vi "Aquire Thermal Data.vi"(8 "error in (no error)":errorcluster, 10 "AI Aquisition Time(s)":dbl, 11 "Recipe Process in":refnum<class "Recipe Process.lvclass">) -> (0 "error out":errorcluster, 3 "Recipe Process out":refnum<class "Recipe Process.lvclass">)   [LabVIEW 2022 SP3, in "Recipe Process.lvlib" / "Recipe Process.lvclass"]
uses:
  Recipe Process.lvclass
  Recipe Process.lvclass/Recipe Process.ctl
  Camera/Camera Controller/Camera Controller.lvclass
  IO Monitor/DAQ API/DAQ API.lvclass
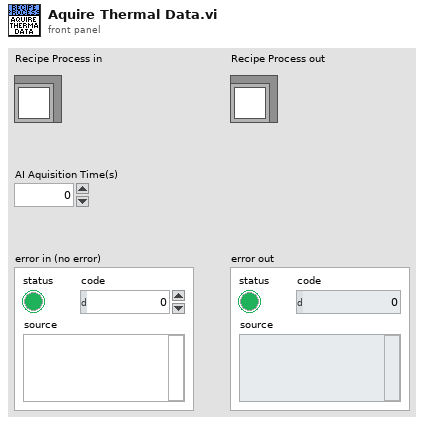
[diagram p1: front panel]
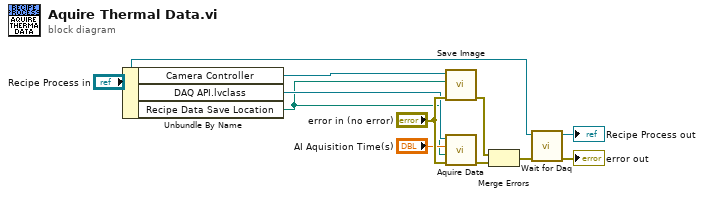
[diagram p0: block diagram]
diagram:
  n1 = Unbundle By Name("Recipe Process in") -> ("Camera Controller"=w2:refnum<class "Camera Controller.lvclass">, "DAQ API.lvclass"=w3:refnum<class "DAQ API.lvclass">, "Recipe Data Save Location"=w1:path)
  n2 = call-dynamic "Save Image.vi"("error in (no error)"="error in (no error)", "Path"=w1, "Camera Controller in"=w2) -> ("error out"=w6:errorcluster)  [unwired: 7 in, 1 out]
  n3 = call-dynamic "Aquire Data.vi"("error in (no error)"="error in (no error)", "Data Save Location"=w1, "Aqusition Time (s)"="AI Aquisition Time(s)", "Aquire Data in"=w3) -> ("error out"=w7:errorcluster)  [unwired: 6 in, 1 out]
  n4 = Merge Errors(w6, w7) -> (w9:errorcluster)
  n5 = call "Wait for Daq.vi"("error in (no error)"=w9, "Recipe Process in"="Recipe Process in") -> ("error out"=→"error out":errorcluster, "Recipe Process out"=→"Recipe Process out":refnum<class "Recipe Process.lvclass">)  [unwired: 8 in]
